vi "Export Mappings.vi"(8 "error in (no error)":errorcluster, 11 "Loop Data":T1) -> (0 "error out":errorcluster)   [LabVIEW 2016, in "System Mapping Tool.lvlib"]
uses:
  System Mapping Tool.lvlib
  TypeDefs/Loop Data.ctl
  TypeDefs/UI Refs.ctl
  NationalInstruments.VeriStand.SystemDefinitionAPI
  NationalInstruments.VeriStand.SystemStorageUI
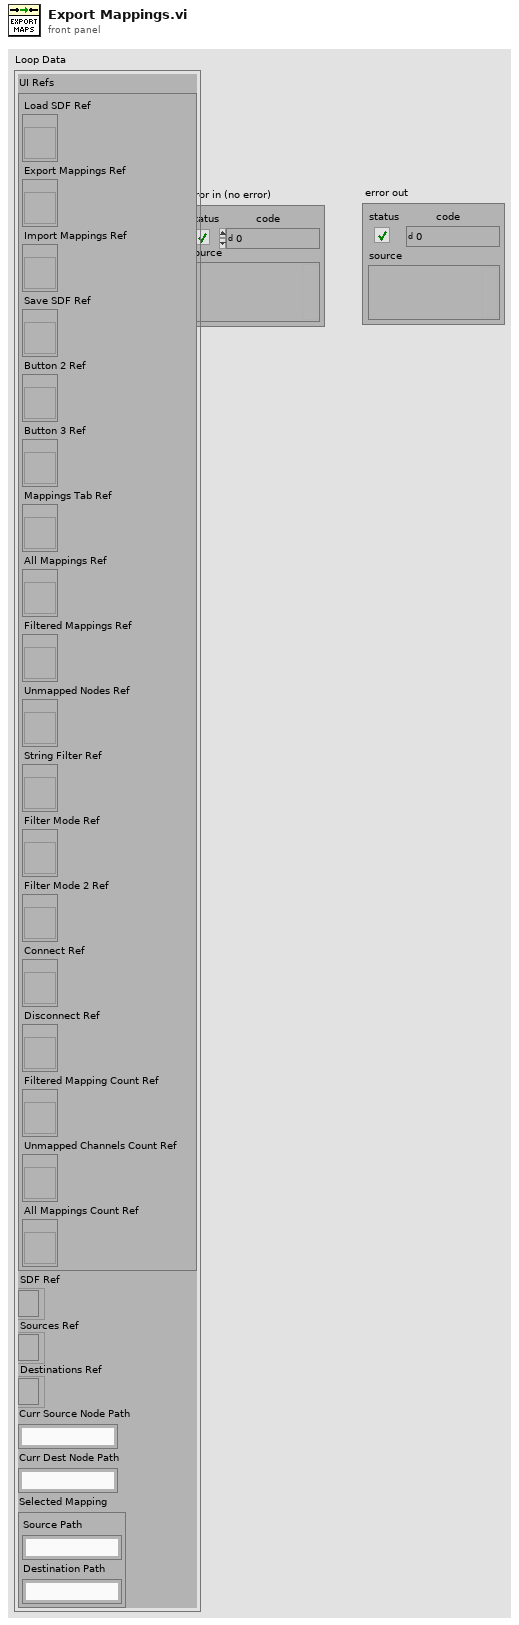
[diagram p1: front panel]
types:
  T1 = typedef "System Mapping Tool.lvlib/Loop Data.ctl" = cluster{"UI Refs":T2, "SDF Ref":refnum<k24>, "Sources Ref":refnum<k24>, "Destinations Ref":refnum<k24>, "Curr Source Node Path":string, "Curr Dest Node Path":string, "Selected Mapping":cluster{"Source Path":string, "Destination Path":string}}
  T2 = typedef "System Mapping Tool.lvlib/UI Refs.ctl" = cluster{"Load SDF Ref":refnum<vi>, "Export Mappings Ref":refnum<vi>, "Import Mappings Ref":refnum<vi>, "Save SDF Ref":refnum<vi>, "Button 2 Ref":refnum<vi>, "Button 3 Ref":refnum<vi>, "Mappings Tab Ref":refnum<vi>, "All Mappings Ref":refnum<vi>, "Filtered Mappings Ref":refnum<vi>, "Unmapped Nodes Ref":refnum<vi>, "String Filter Ref":refnum<vi>, "Filter Mode Ref":refnum<vi>, "Filter Mode 2 Ref":refnum<vi>, "Connect Ref":refnum<vi>, "Disconnect Ref":refnum<vi>, "Filtered Mapping Count Ref":refnum<vi>, "Unmapped Channels Count Ref":refnum<vi>, "All Mappings Count Ref":refnum<vi>}
  T3 = enum32{"All System Mappings", "Filtered Mappings by Node", "Unmapped Channels by Node"}
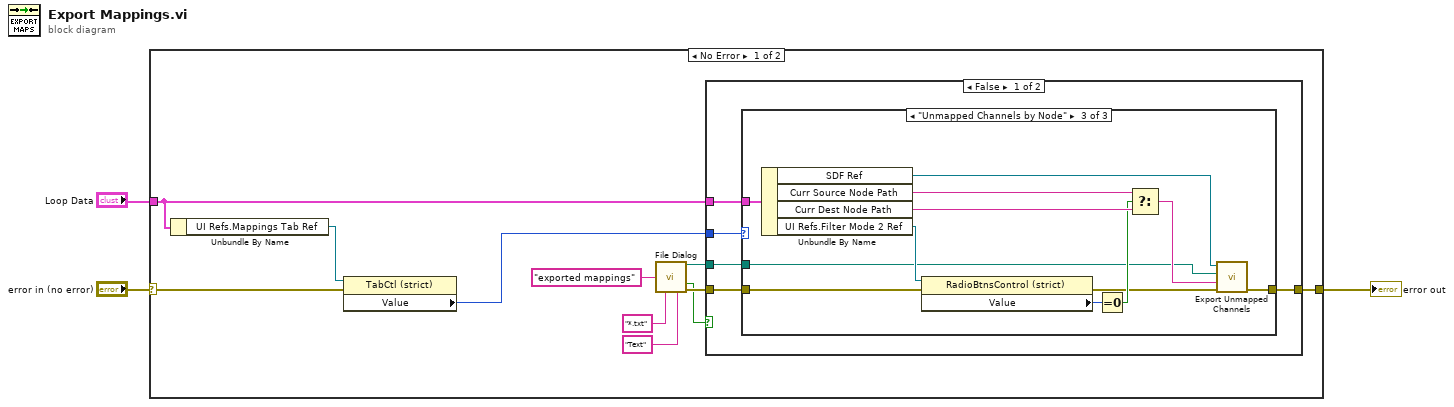
[diagram p0: block diagram]
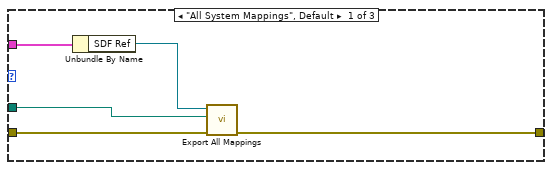
[diagram p2: hidden frame]
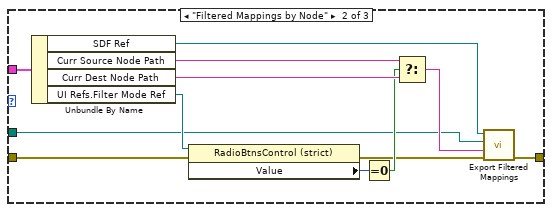
[diagram p3: hidden frame]
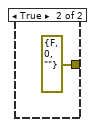
[diagram p4: hidden frame]
diagram:
  n1 = case shown="No Error" "error in (no error)" {
    selector: "error in (no error)" -> [w14 w50]
    tunnel: [w8 w50] -> w2
    tunnel: "Loop Data" -> [w5 _]
    frame No Error {
      n2 = Unbundle By Name(w5) -> ("UI Refs.Mappings Tab Ref"=w13:refnum<vi>)
      n3 = property class="TabCtl (strict)"(reference=w13, error in=w14) -> ("Value"=w4:T3)  [unwired: 2 out]
      n4 = call "File Dialog"("default name"="exported mappings", "pattern (all files)"="*.txt", "pattern label"="Text") -> ("selected path"=w6:path, "cancelled"=w7:bool, "error out"=w9:errorcluster)  [unwired: 9 in, 1 out]
      n5 = case shown="False" w7 {
        tunnel: w9 -> [w19 _]
        tunnel: [w17 errorcluster {"status"=FALSE, "code"=0, "source"=""} ("error out")] -> w8
        tunnel: w4 -> [w18 _]
        tunnel: w6 -> [w16 _]
        tunnel: w5 -> [w15 _]
        frame False {
          n6 = case shown="\"Unmapped Channels by Node\"" w18 {
            tunnel: w19 -> [w24 w35 w47]
            tunnel: [w23 w25 w37] -> w17
            tunnel: w16 -> [w22 w26 w38]
            tunnel: w15 -> [w21 w36 w48]
            frame "All System Mappings", Default {
              n7 = Unbundle By Name(w21) -> ("SDF Ref"=w20:refnum<k24>)
              n8 = call "Export All Mappings.vi"("error in (no error)"=w24, "Path"=w22, "SDF Ref"=w20) -> ("error out"=w23:errorcluster)  [unwired: 8 in]
            }
            frame "Filtered Mappings by Node" {
              n9 = Unbundle By Name(w36) -> ("SDF Ref"=w27:refnum<k24>, "Curr Source Node Path"=w31:string, "Curr Dest Node Path"=w32:string, "UI Refs.Filter Mode Ref"=w34:refnum<vi>)
              n10 = property class="RadioBtnsControl (strict)"(reference=w34, error in=w35) -> (error out=w29:errorcluster, "Value"=w33:enum32{"By Source", "By Destination"})  [unwired: 1 out]
              n11 = Equal To 0?(x=w33) -> (x = 0?=w30:bool)
              n12 = Select(t=w31, s=w30, f=w32) -> (s? t:f=w28:string)
              n13 = call "Export Filtered Mappings.vi"("error in (no error)"=w29, "Filtered Node"=w28, "Path"=w26, "SDF Ref"=w27) -> ("error out"=w25:errorcluster)  [unwired: 7 in]
            }
            frame "Unmapped Channels by Node" {
              n14 = Unbundle By Name(w48) -> ("SDF Ref"=w39:refnum<k24>, "Curr Source Node Path"=w43:string, "Curr Dest Node Path"=w44:string, "UI Refs.Filter Mode 2 Ref"=w46:refnum<vi>)
              n15 = property class="RadioBtnsControl (strict)"(reference=w46, error in=w47) -> (error out=w41:errorcluster, "Value"=w45:enum32{"By Source", "By Destination"})  [unwired: 1 out]
              n16 = Equal To 0?(x=w45) -> (x = 0?=w42:bool)
              n17 = Select(t=w43, s=w42, f=w44) -> (s? t:f=w40:string)
              n18 = call "Export Unmapped Channels.vi"("error in (no error)"=w41, "Filtered Node"=w40, "Path"=w38, "SDF Ref"=w39) -> ("error out"=w37:errorcluster)  [unwired: 7 in]
            }
          }
        }
        frame True {
        }
      }
    }
    frame Error {
    }
  }
  "error out" <- w2
